vi "曲线对齐sub.vi"(10 "测量":cluster{dbl[], dbl[]}, 11 "理论":cluster{dbl[], dbl[]}) -> (1 "数据更改":bool, 2 "实测":cluster{dbl[], dbl[]}, 3 "理论":cluster{dbl[], dbl[]})   [LabVIEW 2015]
panel:
  out "退出":bool
  out "确认操作":bool
  in  "取消":bool
  in  "幅值修正":dbl
  in  "确定移动":bool
  out "输出簇 4":cluster{"x":dbl[], "y":dbl[]}
  out "输出簇 3":cluster{"x":dbl[], "y":dbl[]}
  out "输出簇 2":cluster{"x":dbl[], "y":dbl[]}
  out "输出簇1":cluster{"x":dbl[], "y":dbl[]}
  out "Position.X":dbl
  out "min(x,y)":dbl
  out "max(x,y)":dbl
  in  "动作":enum16{"设置范围", "设置峰值", "移动峰值"}(ring)
  in  "确定":bool
  out "XY图":cluster{dbl[], dbl[]}[](graph)
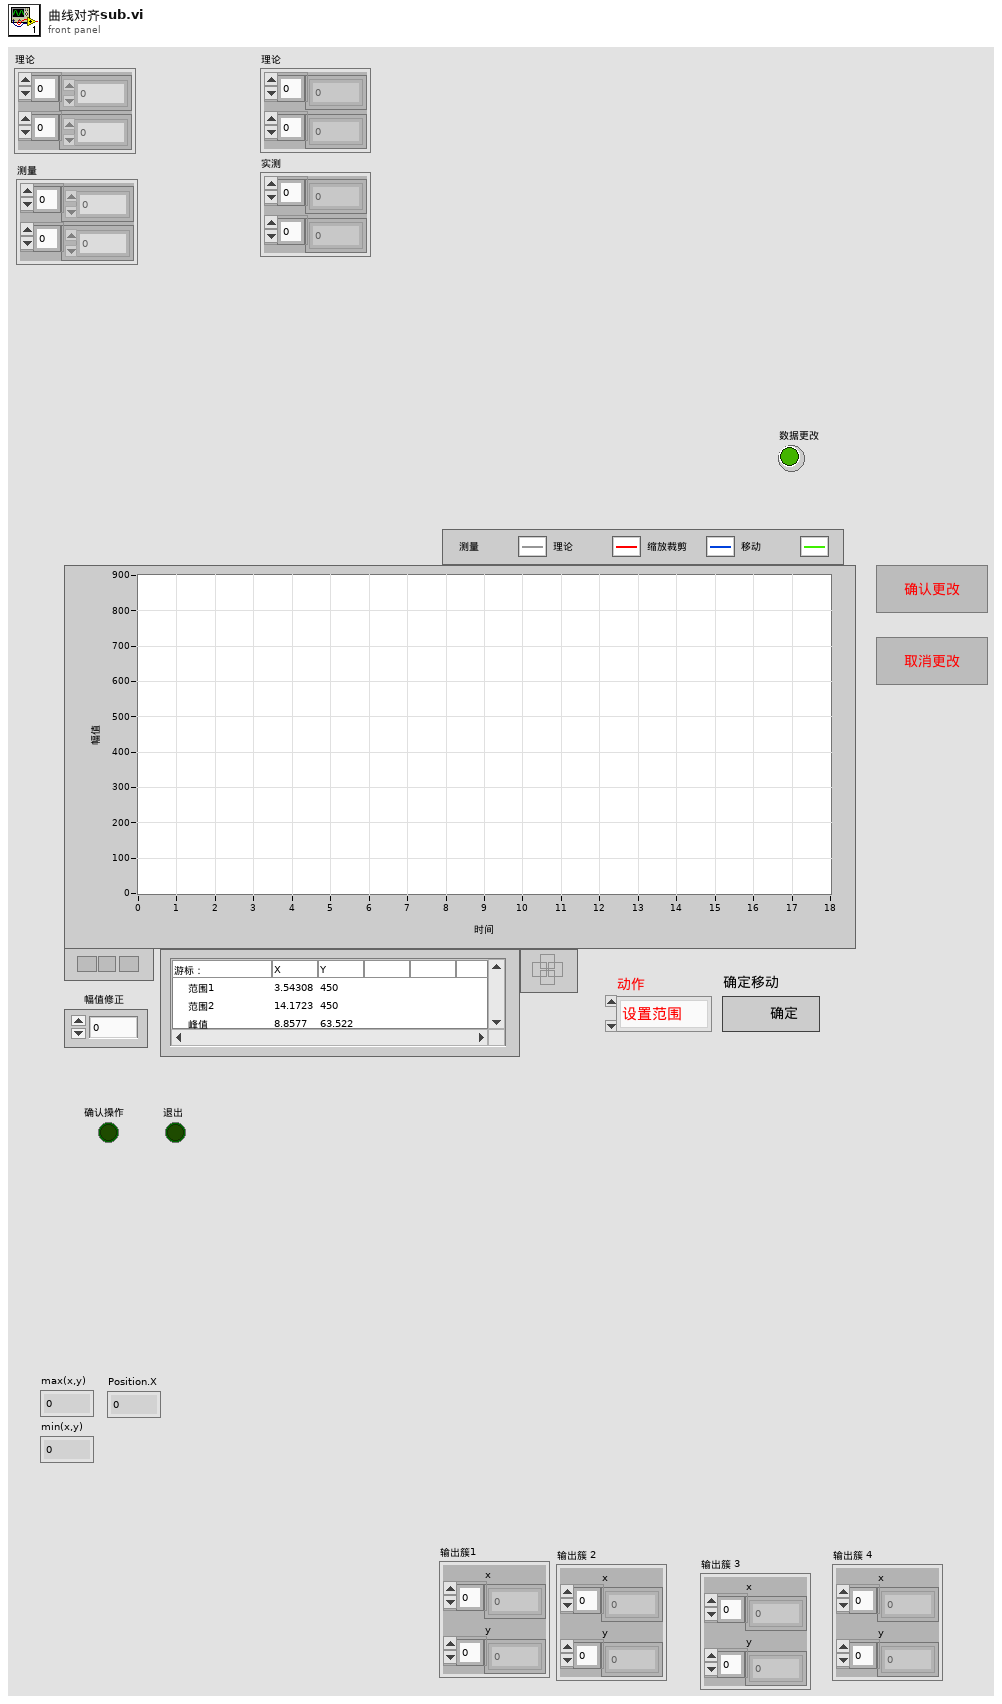
[diagram p1: front panel]
types:
  T1 = typedef "LVCursorListTypeDef.ctl" = cluster{"Name":string, "Color":u32, "Style":u8, "Point Style":u8, "Name Visible":bool, "Allow Drag":bool, "Cursor Mode":u32, "Plot":i32, "Index":i32, "Position":cluster{"X":dbl, "Y":dbl}, "X Scale":u32, "Y Scale":u32, "Watch Plots":i32[], "Watch All Plots":bool, "Plot Area":i32, "Label Offset":cluster{"X":dbl, "Y":dbl}}[]
  T2 = cluster{"Name":string, "Color":u32, "Style":u8, "Point Style":u8, "Name Visible":bool, "Allow Drag":bool, "Cursor Mode":u32, "Plot":i32, "Index":i32, "Position":cluster{"X":dbl, "Y":dbl}, "X Scale":u32, "Y Scale":u32, "Watch Plots":i32[], "Watch All Plots":bool, "Plot Area":i32, "Label Offset":cluster{"X":dbl, "Y":dbl}}
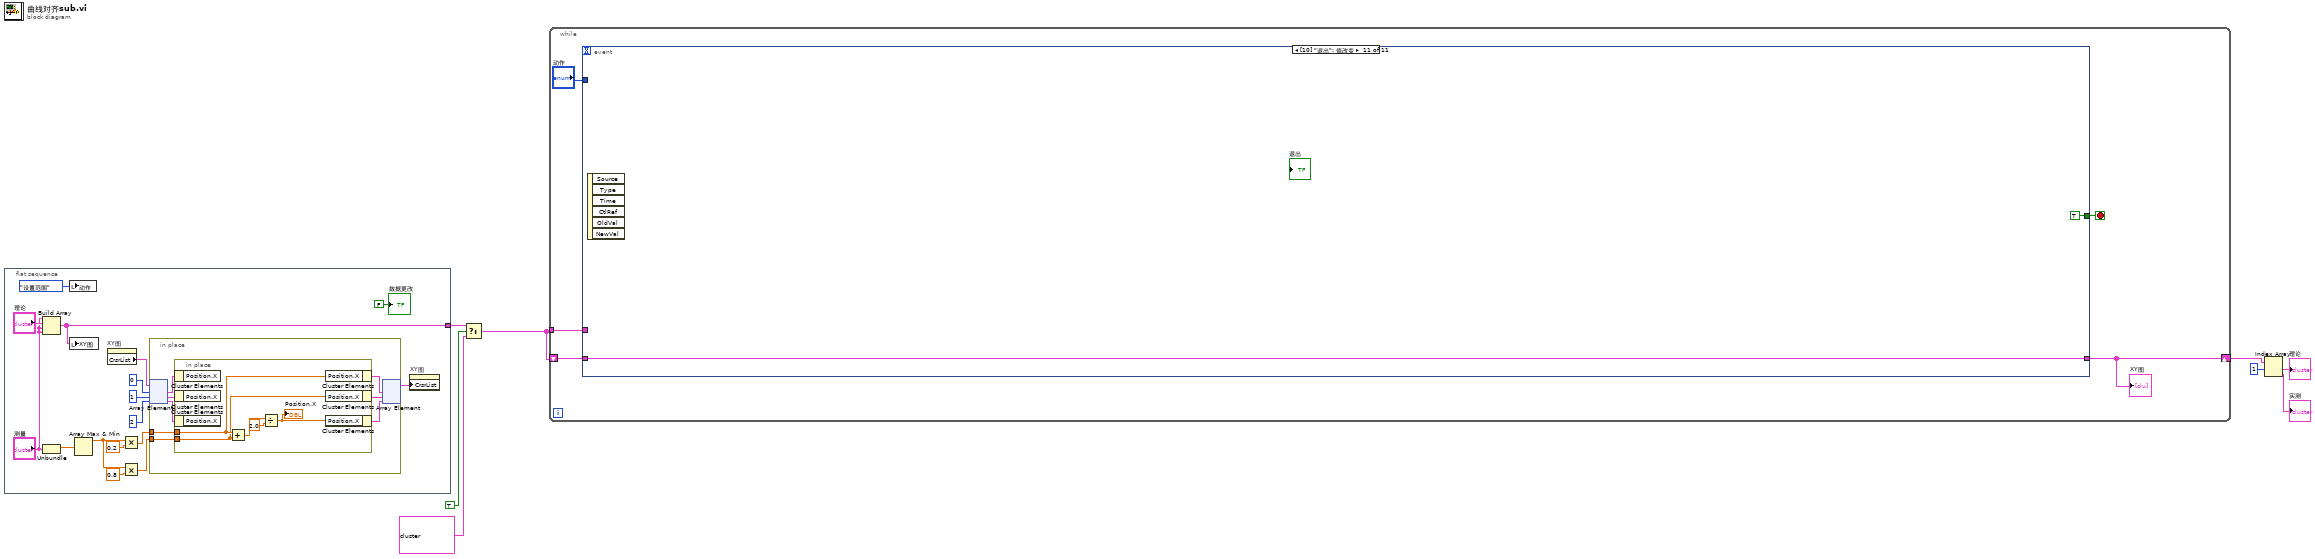
[diagram p0: block diagram]
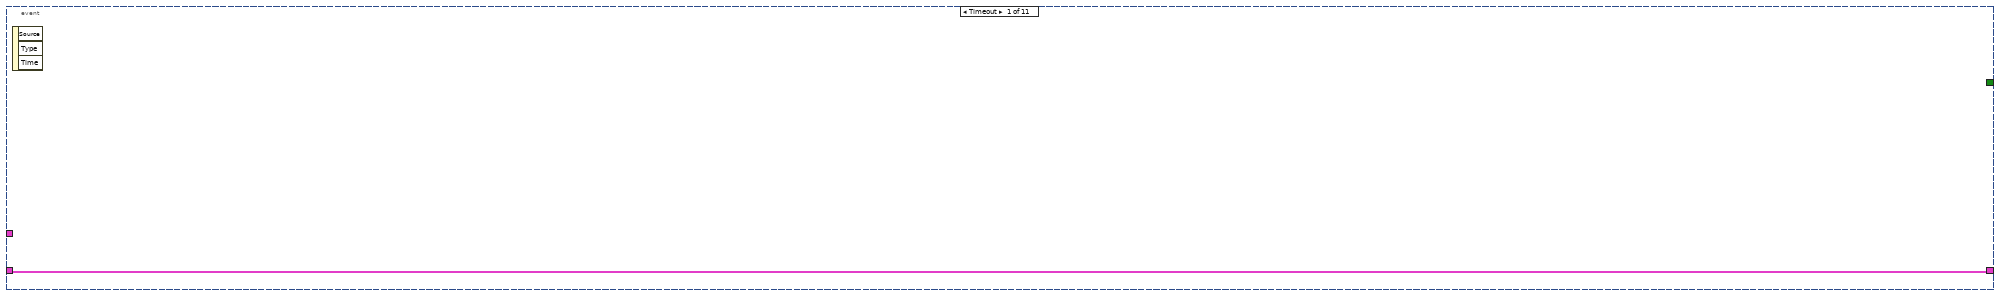
[diagram p2: hidden frame]
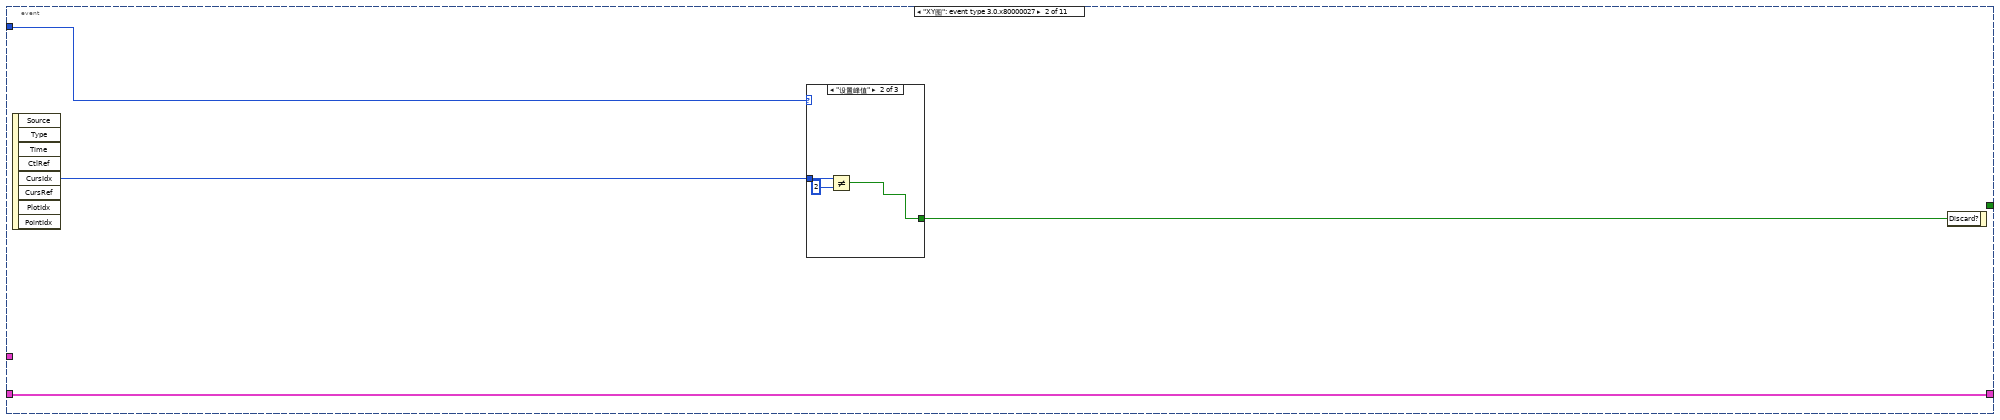
[diagram p3: hidden frame]
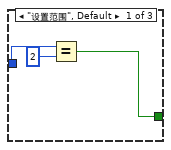
[diagram p4: hidden frame]
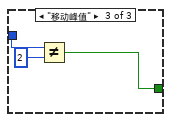
[diagram p5: hidden frame]
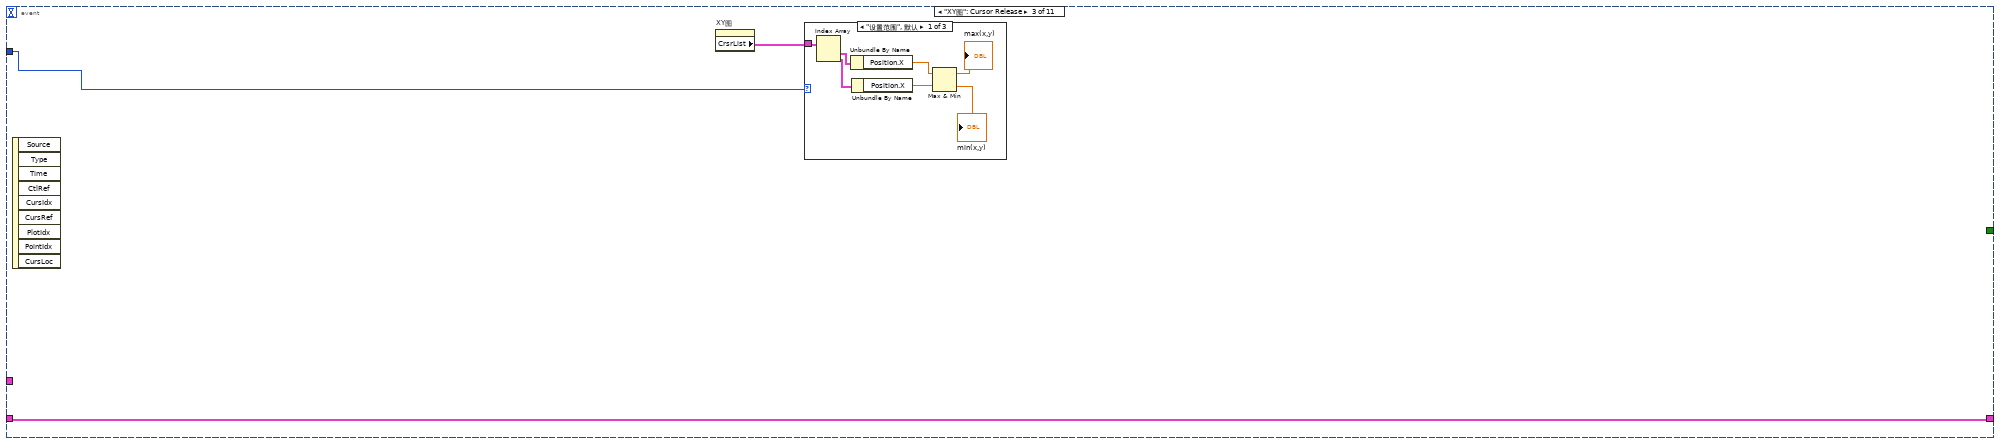
[diagram p6: hidden frame]
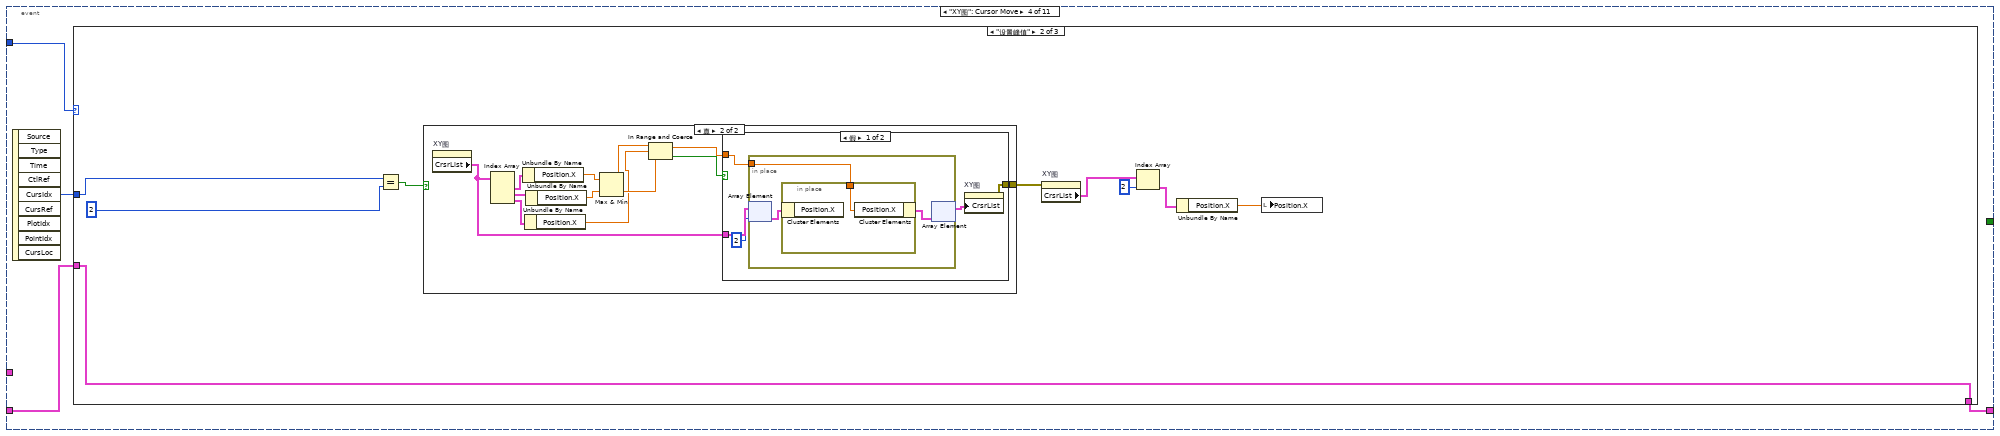
[diagram p9: hidden frame]
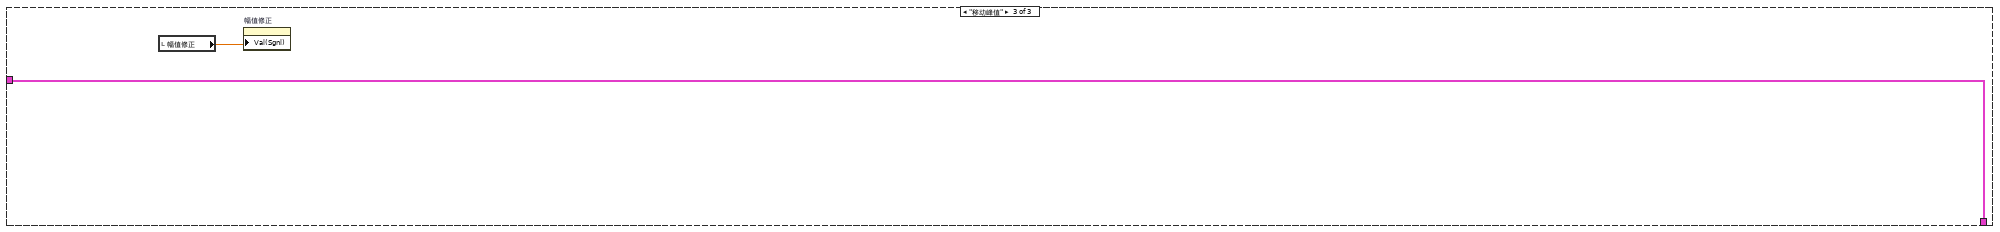
[diagram p13: hidden frame]
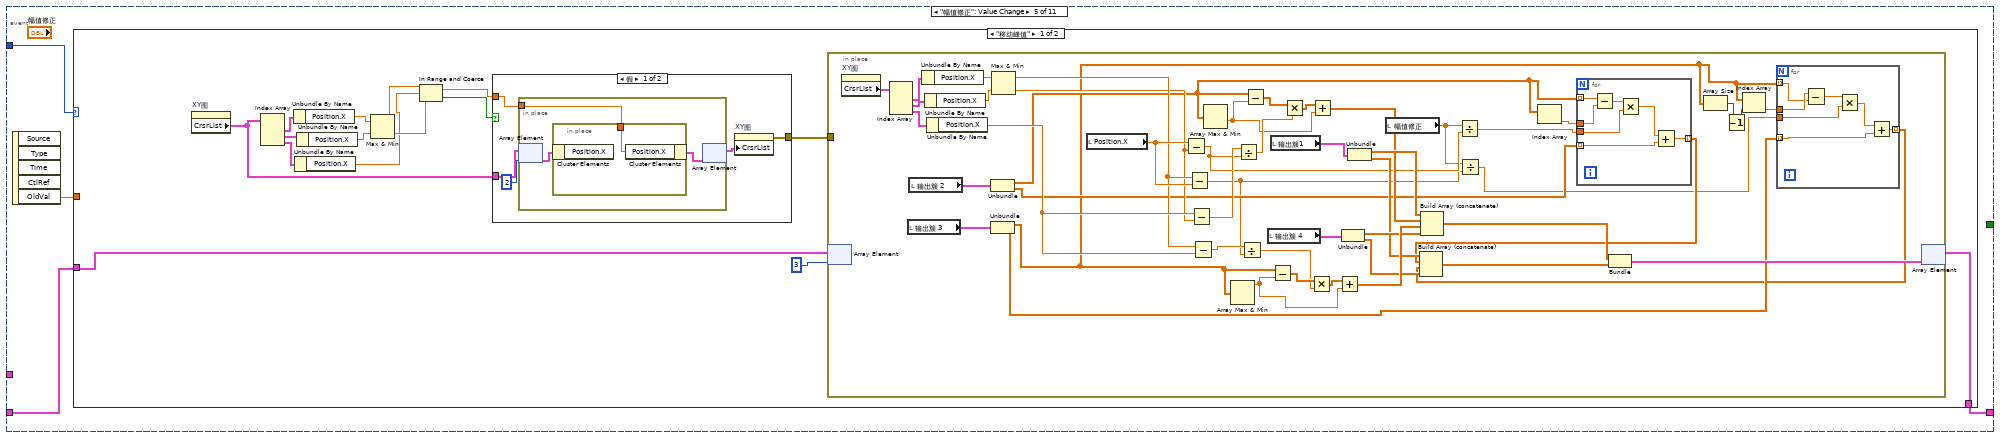
[diagram p14: hidden frame]
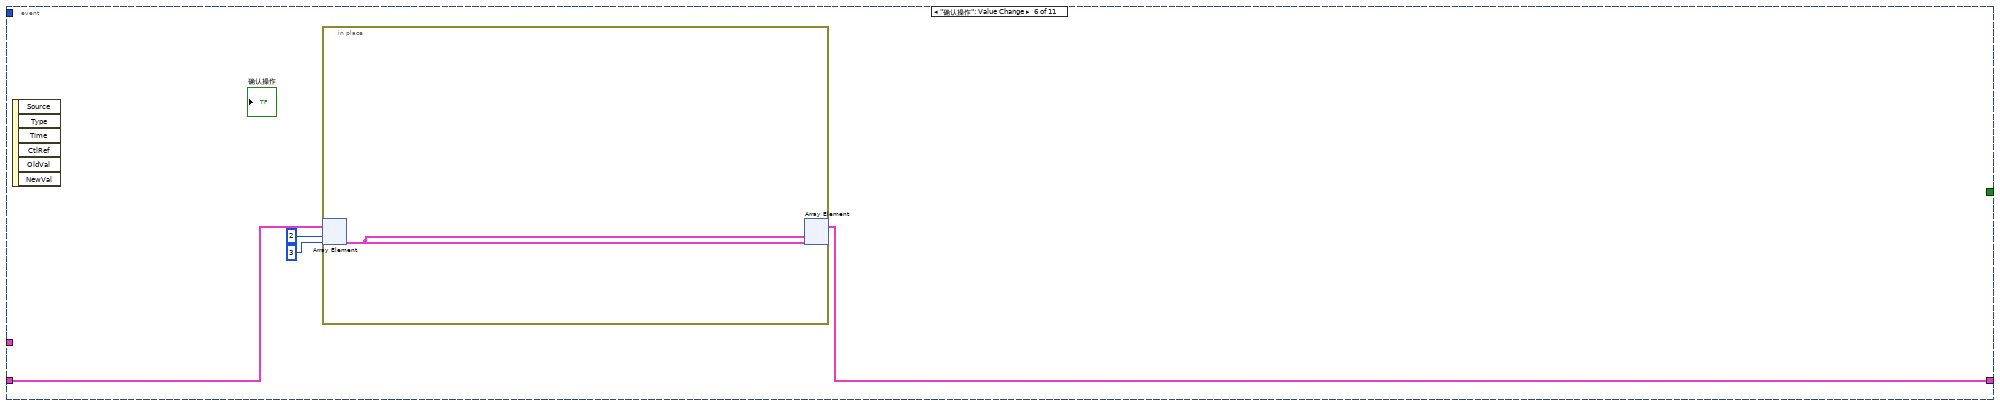
[diagram p17: hidden frame]
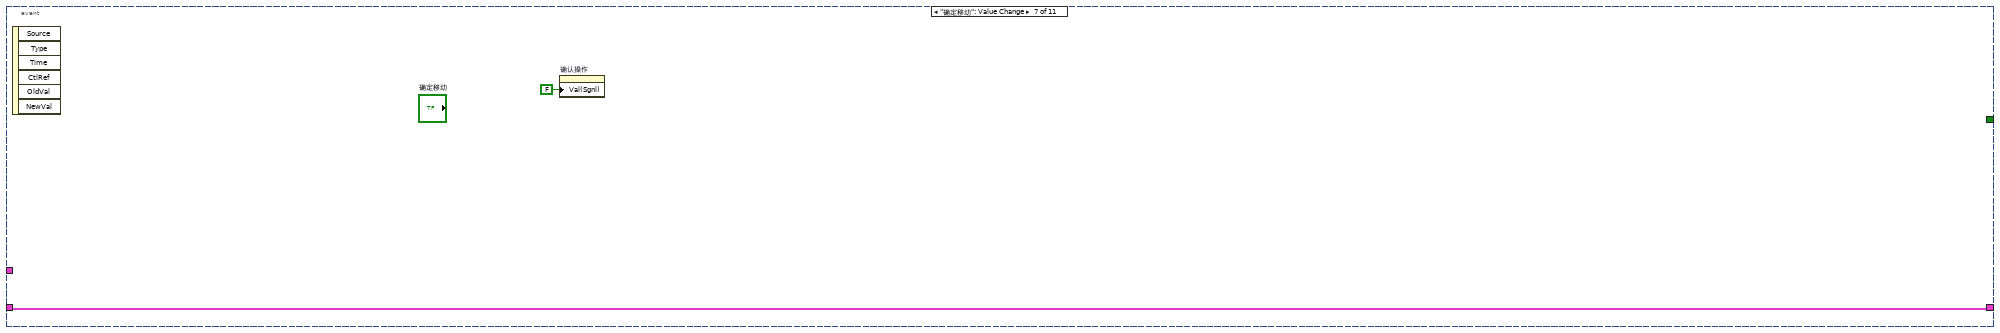
[diagram p18: hidden frame]
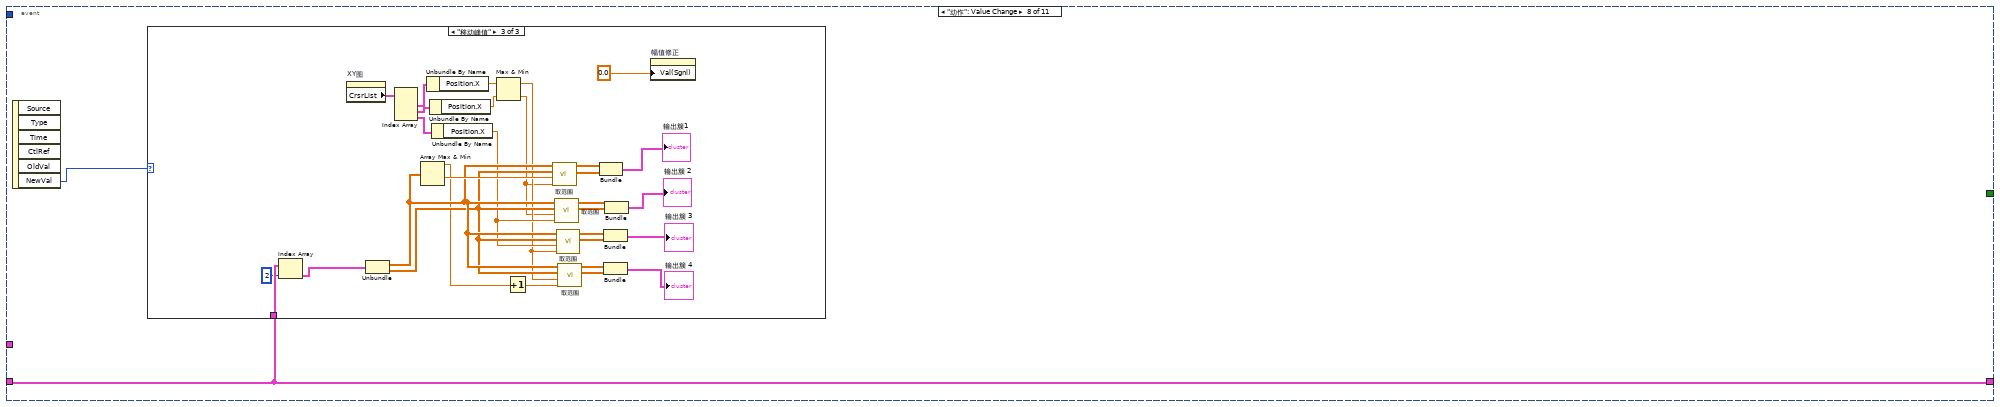
[diagram p19: hidden frame]
diagram:
  n1 = flat-sequence {
    tunnel: [w23] -> w4
    frame #0 {
      n2 = Build Array("测量", "理论", "测量", "测量") -> (w23:cluster{dbl[], dbl[]}[])
      n3 = Unbundle("测量") -> (w20:dbl[])  [unwired: 1 out]
      n4 = local write "动作"(enum16{"设置范围", "设置峰值", "移动峰值"}."设置范围" ("动作")) -> ()
      n5 = local write "XY图"(w23) -> ()
      n6 = Array Max & Min(array=w20) -> (max value=w19:dbl)  [unwired: 3 out]
      n7 = property on="XY图" class="XYGraph (严格)"() -> ("CrsrList"=w16:T1)  [unwired: 2 in, 2 out]
      n8 = Multiply(x=w19, y=0.2) -> (x*y=w12:dbl)
      n9 = Multiply(x=w19, y=0.8) -> (x*y=w11:dbl)
      n10 = in-place {
        in-place-border: w12 -> [w28]
        in-place-border: w11 -> [w27]
        n11 = in-place-array #1(w16, 0, 1, 2) -> (w32:T2, w31:T2, w26:T2)
        n12 = in-place {
          in-place-border: w28 -> [w37]
          in-place-border: w27 -> [w36]
          n13 = in-place-cluster #2(w32) -> ()  [unwired: 1 out]
          n14 = in-place-cluster #3(w31) -> ()  [unwired: 1 out]
          n15 = in-place-cluster #4(w26) -> ()  [unwired: 1 out]
          n16 = Add(x=w37, y=w36) -> (x+y=w35:dbl)
          n17 = Divide(x=w35, y=2.0) -> (x/y=w33:dbl)
          "Position.X" <- w33
          n18 = in-place-cluster #2("Position.X"=w37) -> (w30:T2)
          n19 = in-place-cluster #3("Position.X"=w36) -> (w29:T2)
          n20 = in-place-cluster #4("Position.X"=w33) -> (w25:T2)
        }
        n21 = in-place-array #1(w30, w29, w25) -> (w13:T1)  [unwired: 3 out]
      }
      n22 = property on="XY图" class="XYGraph (严格)"("CrsrList"=w13) -> ()  [unwired: 2 in, 2 out]
      "数据更改" <- FALSE ("数据更改")
    }
  }
  n23 = Select(t=w4, s=TRUE, f=cluster{dbl[], dbl[]}[] [{array[779 elements], array[779 elements]}, {[0.0, 0.744, 1.392, 2.112, 2.725, 3.073, 4.416, 4.788, 5.52, 6.804, 7.249, 7.801, 9.66, 10.489, 10.944, 11.341, 11.676, 11.988, 14.628, 15.288, 16.056, 16.821, 17.653], [0.0, 84.0, 194.0, 425.0, 493.0, 442.0, 431.0, 313.0, 395.0, 307.0, 263.0, 367.0, 309.0, 272.0, 259.0, 307.0, 310.0, 322.0, 408.0, 578.0, 803.0, 596.0, 0.0]}, {array[779 elements], array[779 elements]}, {array[779 elements], array[779 elements]}] ("XY图")) -> (s? t:f=w3:cluster{dbl[], dbl[]}[])
  n24 = while {
    shift-right: [w39] -> w7
    shift-left: w3 -> [w40]
    tunnel: w3 -> [w38]
    stop <- w42 stop-if-true
    n25 = event shown="[10] \"退出\": 值改变" {
      selector: _ -> [_ _ _ _ _ _ _ _ _ _ _]
      dyn-events: _ -> [_ _ _ _ _ _ _ _ _ _ _]
      timeout: _ -> [_ _ _ _ _ _ _ _ _ _ _]
      tunnel: [_ _ _ _ _ _ _ _ _ _ TRUE] -> w42
      tunnel: "动作" -> [_ w45 w59 w70 w107 _ _ _ _ _ _]
      tunnel: w40 -> [w43 w44 w58 w68 w105 w197 w201 w202 w253 _ w258]
      tunnel: [w43 w44 w58 w67 w104 w196 w201 w202 w253 w256 w258] -> w39
      tunnel: w38 -> [_ _ _ _ _ _ _ _ _ w256 _]
      event Timeout {
        n26 = event-data() -> ()  [unwired: 1 in, 3 out]
      }
      event "XY图": event type 3.0.x80000027 {
        n27 = event-data() -> ("CursIdx"=w47:i32)  [unwired: 1 in, 7 out]
        n28 = case shown="\"设置峰值\"" w45 {
          tunnel: w47 -> [w50 w53 w56]
          tunnel: [w48 w51 w54] -> w46
          frame "设置范围", Default {
            n29 = Equal?(x=w50, y=2) -> (x = y?=w48:bool)
          }
          frame "设置峰值" {
            n30 = Not Equal?(x=w53, y=2) -> (x != y?=w51:bool)
          }
          frame "移动峰值" {
            n31 = Not Equal?(x=w56, y=2) -> (x != y?=w54:bool)
          }
        }
        n32 = event-data("Discard?"=w46) -> ()  [unwired: 1 in, 1 out]
      }
      event "XY图": Cursor Release {
        n33 = event-data() -> ()  [unwired: 1 in, 9 out]
        n34 = property on="XY图" class="XYGraph (严格)"() -> ("CrsrList"=w57:T1)  [unwired: 2 in, 2 out]
        n35 = case shown="\"设置范围\", 默认" w59 {
          tunnel: w57 -> [w60 _ _]
          frame "设置范围", Default {
            n36 = Index Array(array=w60) -> (element #1=w66:T2, element #2=w65:T2)  [unwired: 2 in]
            n37 = Unbundle By Name(w66) -> ("Position.X"=w64:dbl)
            n38 = Unbundle By Name(w65) -> ("Position.X"=w63:dbl)
            n39 = Max & Min(x=w64, y=w63) -> (max(x,y)=→"max(x,y)":dbl, min(x,y)=→"min(x,y)":dbl)
          }
          frame "设置峰值" {
          }
          frame "移动峰值" {
          }
        }
      }
      event "XY图": Cursor Move {
        n40 = event-data() -> ("CursIdx"=w69:i32)  [unwired: 1 in, 8 out]
        n41 = case shown="\"设置峰值\"" w70 {
          tunnel: w69 -> [_ w80 _]
          tunnel: w68 -> [w71 w73 w102]
          tunnel: [w71 w73 w102] -> w67
          frame "设置范围", Default {
          }
          frame "设置峰值" {
            n42 = Equal?(x=w80, y=2) -> (x = y?=w78:bool)
            n43 = case shown="真" w78 {
              tunnel: [_ w81] -> w74
              frame False {
              }
              frame True {
                n44 = property on="XY图" class="XYGraph (严格)"() -> ("CrsrList"=w82:T1)  [unwired: 2 in, 2 out]
                n45 = Index Array(array=w82) -> (element #1=w91:T2, element #2=w90:T2, element #3=w92:T2)  [unwired: 3 in]
                n46 = Unbundle By Name(w91) -> ("Position.X"=w89:dbl)
                n47 = Unbundle By Name(w92) -> ("Position.X"=w85:dbl)
                n48 = Unbundle By Name(w90) -> ("Position.X"=w88:dbl)
                n49 = Max & Min(x=w89, y=w88) -> (max(x,y)=w87:dbl, min(x,y)=w86:dbl)
                n50 = In Range and Coerce(upper limit=w87, x=w85, lower limit=w86) -> (coerced(x)=w83:dbl, In Range?=w84:bool)
                n51 = case shown="假" w84 {
                  tunnel: w83 -> [w95 _]
                  tunnel: w82 -> [w97 _]
                  tunnel: [w93 _] -> w81
                  frame False {
                    n52 = in-place {
                      in-place-border: w95 -> [w99]
                      n53 = in-place-array #5(w97, 2) -> (w100:T2)
                      n54 = in-place {
                        in-place-border: w99 -> [w101]
                        n55 = in-place-cluster #6(w100) -> ()  [unwired: 1 out]
                        n56 = in-place-cluster #6("Position.X"=w101) -> (w98:T2)
                      }
                      n57 = in-place-array #5(w98) -> (w94:T1)  [unwired: 1 out]
                    }
                    n58 = property on="XY图" class="XYGraph (严格)"("CrsrList"=w94) -> (error out=w93:errorcluster)  [unwired: 2 in, 1 out]
                  }
                  frame True {
                  }
                }
              }
            }
            n59 = property on="XY图" class="XYGraph (严格)"(error in=w74) -> ("CrsrList"=w77:T1)  [unwired: 1 in, 2 out]
            n60 = Index Array(array=w77, index=2 ("索引")) -> (element=w75:T2)
            n61 = Unbundle By Name(w75) -> ("Position.X"=w72:dbl)
            n62 = local write "Position.X"(w72) -> ()
          }
          frame "移动峰值" {
            n63 = local read "幅值修正"() -> (w103:dbl)
            n64 = property on="幅值修正" class="DigNum (严格)"("Val(Sgnl)"=w103) -> ()  [unwired: 2 in, 2 out]
          }
        }
      }
      event "幅值修正": Value Change {
        n65 = event-data() -> ("OldVal"=w106:dbl)  [unwired: 1 in, 4 out]
        n66 = case shown="\"移动峰值\"" w107 {
          tunnel: w106 -> [_ _]
          tunnel: w105 -> [w122 w194]
          tunnel: [w108 w194] -> w104
          frame "移动峰值" {
            n67 = property on="XY图" class="XYGraph (严格)"() -> ("CrsrList"=w110:T1)  [unwired: 2 in, 2 out]
            n68 = Index Array(array=w110) -> (element #1=w119:T2, element #2=w118:T2, element #3=w120:T2)  [unwired: 3 in]
            n69 = Unbundle By Name(w119) -> ("Position.X"=w117:dbl)
            n70 = Unbundle By Name(w120) -> ("Position.X"=w113:dbl)
            n71 = Unbundle By Name(w118) -> ("Position.X"=w116:dbl)
            n72 = Max & Min(x=w117, y=w116) -> (max(x,y)=w115:dbl, min(x,y)=w114:dbl)
            n73 = In Range and Coerce(upper limit=w115, x=w113, lower limit=w114) -> (coerced(x)=w111:dbl, In Range?=w112:bool)
            n74 = case shown="假" w112 {
              tunnel: w111 -> [w125 _]
              tunnel: w110 -> [w127 _]
              tunnel: [w123 _] -> w109
              frame False {
                n75 = in-place {
                  in-place-border: w125 -> [w129]
                  n76 = in-place-array #7(w127, 2) -> (w130:T2)
                  n77 = in-place {
                    in-place-border: w129 -> [w131]
                    n78 = in-place-cluster #8(w130) -> ()  [unwired: 1 out]
                    n79 = in-place-cluster #8("Position.X"=w131) -> (w128:T2)
                  }
                  n80 = in-place-array #7(w128) -> (w124:T1)  [unwired: 1 out]
                }
                n81 = property on="XY图" class="XYGraph (严格)"("CrsrList"=w124) -> (error out=w123:errorcluster)  [unwired: 2 in, 1 out]
              }
              frame True {
              }
            }
            n82 = in-place {
              in-place-border: w109 -> [_]
              n83 = in-place-array #9(w122, 3) -> ()  [unwired: 1 out]
              n84 = property on="XY图" class="XYGraph (严格)"() -> ("CrsrList"=w179:T1)  [unwired: 2 in, 2 out]
              n85 = Index Array(array=w179) -> (element #1=w178:T2, element #2=w177:T2, element #3=w174:T2)  [unwired: 3 in]
              n86 = local read "输出簇 3"() -> (w161:cluster{"x":dbl[], "y":dbl[]})
              n87 = local read "输出簇 2"() -> (w162:cluster{"x":dbl[], "y":dbl[]})
              n88 = Unbundle By Name(w178) -> ("Position.X"=w176:dbl)
              n89 = Unbundle By Name(w177) -> ("Position.X"=w175:dbl)
              n90 = Unbundle By Name(w174) -> ("Position.X"=w172:dbl)
              n91 = Unbundle(w162) -> ("x"=w145:dbl[], "y"=w143:dbl[])
              n92 = Unbundle(w161) -> ("x"=w139:dbl[], "y"=w136:dbl[])
              n93 = Max & Min(x=w176, y=w175) -> (max(x,y)=w171:dbl, min(x,y)=w170:dbl)
              n94 = local read "Position.X"() -> (w173:dbl)
              n95 = Subtract(x=w173, y=w170) -> (x-y=w134:dbl)
              n96 = Subtract(x=w171, y=w173) -> (x-y=w133:dbl)
              n97 = Subtract(x=w172, y=w170) -> (x-y=w148:dbl)
              n98 = Subtract(x=w171, y=w172) -> (x-y=w147:dbl)
              n99 = Array Max & Min(array=w145) -> (min value=w166:dbl)  [unwired: 3 out]
              n100 = Array Max & Min(array=w139) -> (max value=w160:dbl)  [unwired: 3 out]
              n101 = Divide(x=w148, y=w134) -> (x/y=w168:dbl)
              n102 = Divide(x=w147, y=w133) -> (x/y=w163:dbl)
              n103 = Subtract(x=w145, y=w166) -> (x-y=w169:dbl[])
              n104 = local read "输出簇 4"() -> (w158:cluster{"x":dbl[], "y":dbl[]})
              n105 = local read "输出簇1"() -> (w159:cluster{"x":dbl[], "y":dbl[]})
              n106 = Subtract(x=w139, y=w160) -> (x-y=w164:dbl[])
              n107 = Multiply(x=w169, y=w168) -> (x*y=w167:dbl[])
              n108 = Multiply(x=w164, y=w163) -> (x*y=w165:dbl[])
              n109 = Add(x=w167, y=w166) -> (x+y=w156:dbl[])
              n110 = Add(x=w165, y=w160) -> (x+y=w155:dbl[])
              n111 = Unbundle(w158) -> ("x"=w154:dbl[], "y"=w152:dbl[])
              n112 = Unbundle(w159) -> ("x"=w157:dbl[], "y"=w153:dbl[])
              n113 = local read "幅值修正"() -> (w132:dbl)
              n114 = Build Array (concatenate)(w157, w156, w155, w154) -> (w151:dbl[])
              n115 = Divide(x=w132, y=w134) -> (x/y=w144:dbl)
              n116 = Divide(x=w132, y=w133) -> (x/y=w137:dbl)
              n117 = Index Array(array=w145) -> (element=w146:dbl)  [unwired: 1 in]
              n118 = for {
                tunnel: w145 -> [w193] mode=indexing
                tunnel: w146 -> [w192]
                tunnel: w144 -> [w190]
                tunnel: w143 -> [w188] mode=indexing
                tunnel: [w187] -> w142 mode=indexing
                n119 = Subtract(x=w193, y=w192) -> (x-y=w191:dbl)
                n120 = Multiply(x=w191, y=w190) -> (x*y=w189:dbl)
                n121 = Add(x=w189, y=w188) -> (x+y=w187:dbl)
              }
              n122 = Array Size(array=w139) -> (size(s)=w141:i32)
              n123 = Decrement(x=w141) -> (x-1=w140:i32)
              n124 = Index Array(array=w139, index=w140) -> (element=w138:dbl)
              n125 = for {
                tunnel: w139 -> [w185] mode=indexing
                tunnel: w138 -> [w186]
                tunnel: w137 -> [w183]
                tunnel: w136 -> [w181] mode=indexing
                tunnel: [w180] -> w135 mode=indexing
                n126 = Subtract(x=w186, y=w185) -> (x-y=w184:dbl)
                n127 = Multiply(x=w184, y=w183) -> (x*y=w182:dbl)
                n128 = Add(x=w182, y=w181) -> (x+y=w180:dbl)
              }
              n129 = Build Array (concatenate)(w153, w142, w135, w152) -> (w150:dbl[])
              n130 = Bundle(w151, w150) -> (w149:cluster{dbl[], dbl[]})  [unwired: 1 in]
              n131 = in-place-array #9(w149) -> (w108:cluster{dbl[], dbl[]}[])  [unwired: 1 out]
            }
          }
          frame Default {
          }
        }
      }
      event "确认操作": Value Change {
        n132 = event-data() -> ()  [unwired: 1 in, 6 out]
        n133 = in-place {
          n134 = in-place-array #10(w197, 2, 3) -> (w199:cluster{dbl[], dbl[]})  [unwired: 1 out]
          n135 = in-place-array #10(w199, w199) -> (w196:cluster{dbl[], dbl[]}[])  [unwired: 2 out]
        }
      }
      event "确定移动": Value Change {
        n136 = event-data() -> ()  [unwired: 1 in, 6 out]
        n137 = property on="确认操作" class="Bool (严格)"("Val(Sgnl)"=FALSE ("值(信号)")) -> ()  [unwired: 2 in, 2 out]
      }
      event "动作": Value Change {
        n138 = event-data() -> ("NewVal"=w203:enum16{"设置范围", "设置峰值", "移动峰值"})  [unwired: 1 in, 5 out]
        n139 = case shown="\"移动峰值\"" w203 {
          tunnel: w202 -> [_ _ w227]
          frame "设置范围", Default {
          }
          frame "设置峰值" {
            n140 = case shown="真" TRUE {
              frame False {
              }
              frame True {
                n141 = property on="XY图" class="XYGraph (严格)"() -> ("CrsrList"=w212:T1)  [unwired: 2 in, 2 out]
                n142 = Index Array(array=w212) -> (element #1=w214:T2, element #2=w213:T2)  [unwired: 2 in]
                n143 = Unbundle By Name(w214) -> ("Position.X"=w211:dbl)
                n144 = Unbundle By Name(w213) -> ("Position.X"=w210:dbl)
                n145 = Add(x=w211, y=w210) -> (x+y=w209:dbl)
                n146 = Divide(x=w209, y=2.0) -> (x/y=w205:dbl)
                n147 = local write "Position.X"(w205) -> ()
                n148 = in-place {
                  in-place-border: w205 -> [w215]
                  n149 = in-place-array #11(w212, 2) -> (w217:T2)
                  n150 = in-place {
                    in-place-border: w215 -> [w218]
                    n151 = in-place-cluster #12(w217) -> ()  [unwired: 1 out]
                    n152 = in-place-cluster #12("Position.X"=w218) -> (w216:T2)
                  }
                  n153 = in-place-array #11(w216) -> (w206:T1)  [unwired: 1 out]
                }
                n154 = property on="XY图" class="XYGraph (严格)"("CrsrList"=w206) -> ()  [unwired: 2 in, 2 out]
              }
            }
          }
          frame "移动峰值" {
            n155 = Index Array(array=w227, index=2 ("索引")) -> (element=w225:cluster{dbl[], dbl[]})
            n156 = property on="XY图" class="XYGraph (严格)"() -> ("CrsrList"=w248:T1)  [unwired: 2 in, 2 out]
            n157 = Unbundle(w225) -> (w241:dbl[], w240:dbl[])
            n158 = Index Array(array=w248) -> (element #1=w247:T2, element #2=w246:T2, element #3=w243:T2)  [unwired: 3 in]
            n159 = Array Max & Min(array=w241) -> (max value=w239:dbl, min value=w242:dbl)  [unwired: 2 out]
            n160 = Unbundle By Name(w247) -> ("Position.X"=w245:dbl)
            n161 = Unbundle By Name(w246) -> ("Position.X"=w244:dbl)
            n162 = Unbundle By Name(w243) -> ("Position.X"=w234:dbl)
            n163 = Max & Min(x=w245, y=w244) -> (max(x,y)=w233:dbl, min(x,y)=w232:dbl)
            n164 = Increment(x=w239) -> (x+1=w219:dbl)
            n165 = call "取范围.vi"("max"=w232, "min"=w242, "y"=w240, "x"=w241) -> ("y"=w237:dbl[], "x"=w238:dbl[])  [unwired: 6 in]
            n166 = call "取范围.vi"("max"=w234, "min"=w232, "y"=w240, "x"=w241) -> ("y"=w228:dbl[], "x"=w231:dbl[])  [unwired: 6 in]
            n167 = call "取范围.vi"("max"=w233, "min"=w234, "y"=w240, "x"=w241) -> ("y"=w229:dbl[], "x"=w230:dbl[])  [unwired: 6 in]
            n168 = call "取范围.vi"("max"=w219, "min"=w233, "y"=w240, "x"=w241) -> ("y"=w235:dbl[], "x"=w236:dbl[])  [unwired: 6 in]
            n169 = Bundle("x"=w238, "y"=w237) -> (→"输出簇1":cluster{"x":dbl[], "y":dbl[]})  [unwired: 1 in]
            n170 = Bundle("x"=w230, "y"=w229) -> (→"输出簇 3":cluster{"x":dbl[], "y":dbl[]})  [unwired: 1 in]
            n171 = Bundle("x"=w236, "y"=w235) -> (→"输出簇 4":cluster{"x":dbl[], "y":dbl[]})  [unwired: 1 in]
            n172 = Bundle("x"=w231, "y"=w228) -> (→"输出簇 2":cluster{"x":dbl[], "y":dbl[]})  [unwired: 1 in]
            n173 = property on="幅值修正" class="DigNum (严格)"("Val(Sgnl)"=0.0 ("幅值修正")) -> ()  [unwired: 2 in, 2 out]
          }
        }
      }
      event "确定": Value Change {
        n174 = event-data() -> ()  [unwired: 1 in, 6 out]
        n175 = property on="确认操作" class="Bool (严格)"("Val(Sgnl)"=FALSE ("值(信号)")) -> (error out=w250:errorcluster)  [unwired: 2 in, 1 out]
        n176 = property on="退出" class="Bool (严格)"(error in=w250, "Val(Sgnl)"=FALSE ("值(信号)")) -> ()  [unwired: 1 in, 2 out]
        n177 = local write "数据更改"(TRUE ("数据更改")) -> ()
      }
      event "取消": Value Change; Panel Close {
        n178 = event-data() -> ()  [unwired: 1 in, 3 out]
        n179 = property on="退出" class="Bool (严格)"("Val(Sgnl)"=FALSE ("值(信号)")) -> ()  [unwired: 2 in, 2 out]
        n180 = local write "数据更改"(FALSE ("数据更改")) -> ()
      }
      event "退出": Value Change {
        n181 = event-data() -> ()  [unwired: 1 in, 6 out]
      }
    }
    "XY图" <- w39
  }
  n182 = Index Array(array=w7, index #1=1 ("索引")) -> (element #1=→"理论":cluster{dbl[], dbl[]}, element #2=→"实测":cluster{dbl[], dbl[]})  [unwired: 1 in]
